vi "Two Agilent N6700 Series Configure Voltage.vi"() -> ()   [LabVIEW 2021]
doc: "Configures the power supply's output range on a channel, configures the DC voltage level, channel appears at the output connector and takes a measurement on the output signal and returns the measured value."
uses:
  <instrlib>/Agilent N6700 Series/Agilent N6700 Series.lvlib
panel:
  in  "Vin SMU":refnum<visa-resource-name>
  in  "Vin SMUChannel":string="1"
  in  "Vin Voltage Range":dbl=10.0 format="%^.3e"
  in  "Vin Voltage Level":dbl=5.0 format="%^.3e"
  out "Vin Voltage Measurement":dbl format="%^.3e"
  in  "Vin Behavior":i32(ring) items=["Regulatory Limit", "Trip Limit"]
  in  "Vin Current Limit":dbl=1.0 format="%^.3e"
  in  "error in":errorcluster {"code" format="%.0x"}
  out "error out":errorcluster {"code" format="%.0x"}
  in  "Load Current Limit":dbl=1.0 format="%^.3e"
  in  "Behavior":i32(ring) items=["Regulatory Limit", "Trip Limit"]
  out "Load Voltage Measurement":dbl format="%^.3e"
  in  "Load Voltage Level":dbl=5.0 format="%^.3e"
  in  "Load Voltage Range":dbl=10.0 format="%^.3e"
  in  "Load SMUChannel":string="1"
  in  "Load SMU":refnum<visa-resource-name>
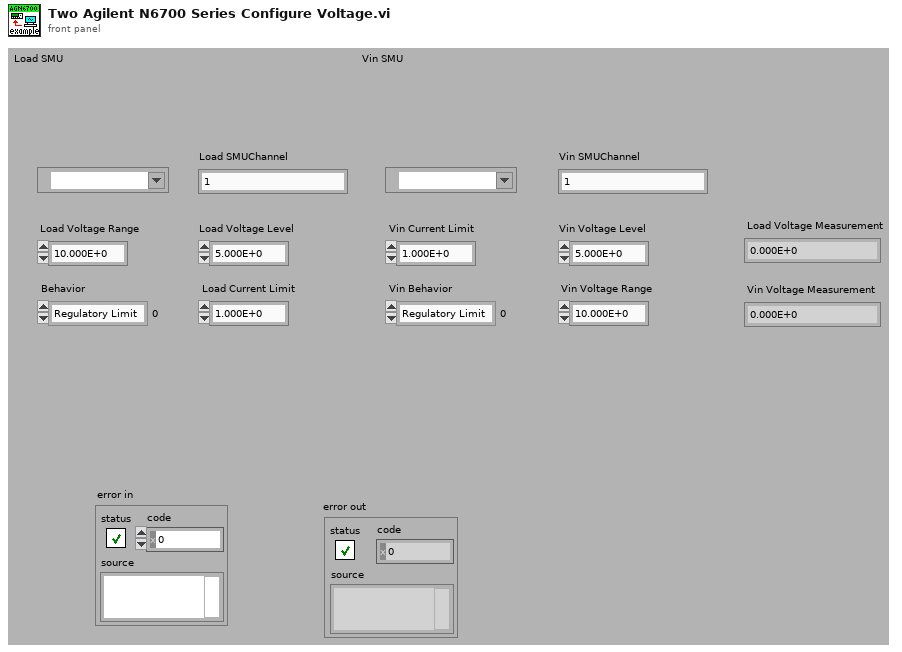
[diagram p1: front panel]
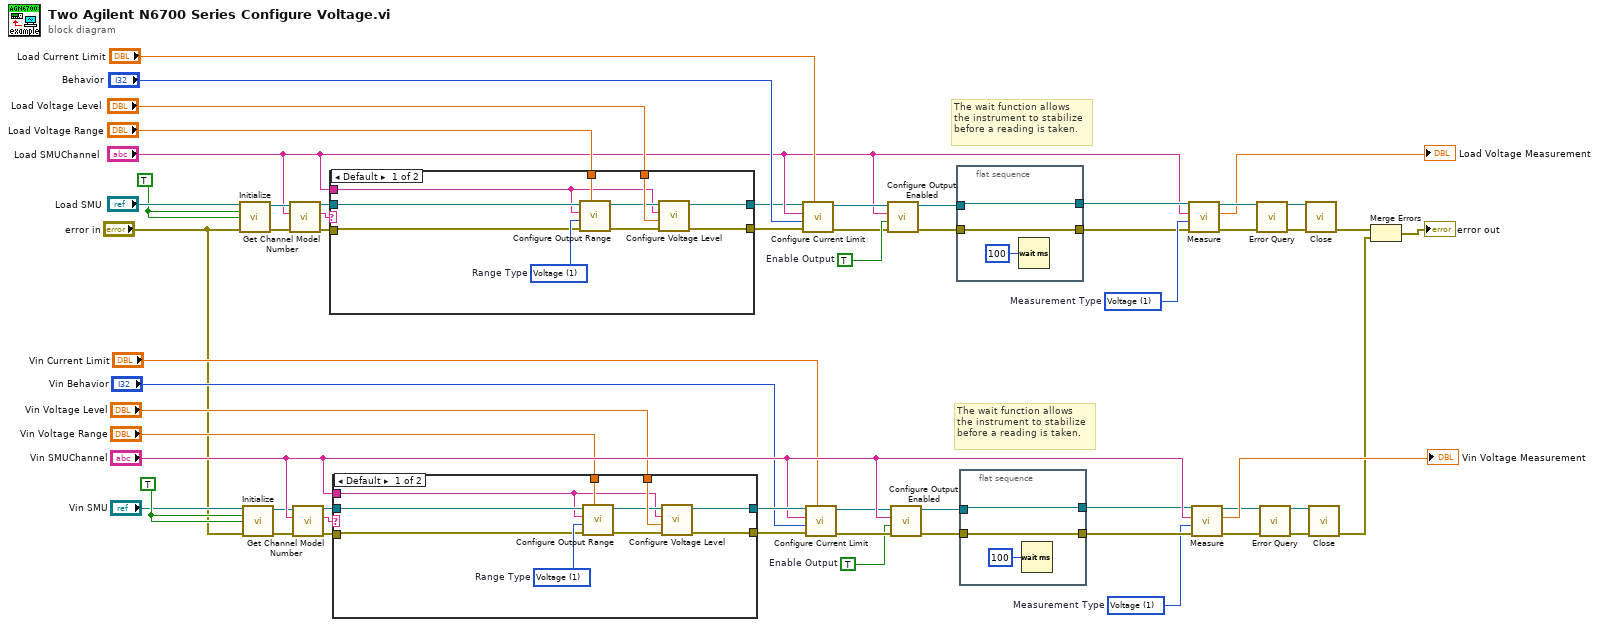
[diagram p0: block diagram]
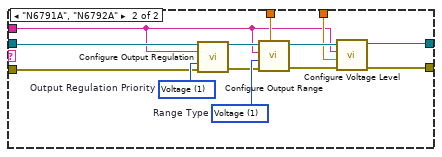
[diagram p2: hidden frame]
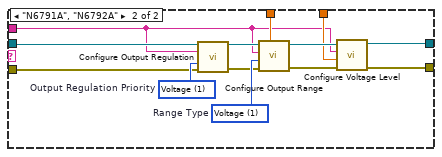
[diagram p3: hidden frame]
diagram:
  w13 = TRUE ("Reset? (T: Yes)")
  w12 = 1 items=["Voltage"=1, "Current"=0]  # Measurement Type
  w11 = TRUE  # Enable Output
  w49 = TRUE ("Reset? (T: Yes)")
  w50 = 1 items=["Voltage"=1, "Current"=0]  # Measurement Type
  w51 = TRUE  # Enable Output
  # "The wait function allows \nthe instrument to stabilize\nbefore a reading is taken."
  # "The wait function allows \nthe instrument to stabilize\nbefore a reading is taken."
  n1 = call <instrlib>:"Initialize.vi"("VISA resource name"="Load SMU", "ID Query? (T: Yes)"=w49, "Reset? (T: Yes)"=w49, "error in (no error)"="error in") -> ("VISA resource name out"=w40:refnum<visa-resource-name>, "error out"=w39:errorcluster)  [unwired: 10 in]
  n2 = call <instrlib>:"Initialize.vi"("VISA resource name"="Vin SMU", "ID Query? (T: Yes)"=w13, "Reset? (T: Yes)"=w13, "error in (no error)"="error in") -> ("VISA resource name out"=w22:refnum<visa-resource-name>, "error out"=w23:errorcluster)  [unwired: 10 in]
  n3 = call <instrlib>:"Get Channel Model Number.vi"("error in (no error)"=w39, "Channel Name (1)"="Load SMUChannel", "VISA resource name"=w40) -> ("error out"=w37:errorcluster, "Model Number"=w36:string, "VISA resource name out"=w38:refnum<visa-resource-name>)  [unwired: 6 in]
  n4 = call <instrlib>:"Get Channel Model Number.vi"("error in (no error)"=w23, "Channel Name (1)"="Vin SMUChannel", "VISA resource name"=w22) -> ("error out"=w25:errorcluster, "Model Number"=w26:string, "VISA resource name out"=w24:refnum<visa-resource-name>)  [unwired: 6 in]
  n5 = case shown="Default" w36 {
    tunnel: "Load Voltage Range" -> [w65 w81]
    tunnel: "Load SMUChannel" -> [w59 w71]
    tunnel: w38 -> [w67 w76]
    tunnel: w37 -> [w66 w75]
    tunnel: "Load Voltage Level" -> [w63 w72]
    tunnel: [w61 w69] -> w33
    tunnel: [w60 w70] -> w32
    frame Default {
      w68 = 1 items=["Voltage"=1, "Current"=0]  # Range Type
      n6 = call <instrlib>:"Configure Output Range.vi"("Range (0.0)"=w65, "error in (no error)"=w66, "Range Type (1: Voltage)"=w68, "Channel Name (1)"=w59, "VISA resource name"=w67) -> ("error out"=w64:errorcluster, "VISA resource name out"=w62:refnum<visa-resource-name>)  [unwired: 5 in]
      n7 = call <instrlib>:"Configure Voltage Level.vi"("error in (no error)"=w64, "Level  (0.0 volts)"=w63, "Channel Name (1)"=w59, "VISA resource name"=w62) -> ("error out"=w61:errorcluster, "VISA resource name out"=w60:refnum<visa-resource-name>)  [unwired: 6 in]
    }
    frame "N6791A", "N6792A" {
      w77 = 1 items=["Voltage"=1, "Current"=0]  # Output Regulation Priority
      w80 = 1 items=["Voltage"=1, "Current"=0]  # Range Type
      n8 = call <instrlib>:"Configure Output Regulation.vi"("VISA resource name"=w76, "Channel Name (1)"=w71, "Output Regulation Priority (1: Voltage)"=w77, "error in (no error)"=w75) -> ("VISA resource name out"=w79:refnum<visa-resource-name>, "error out"=w78:errorcluster)  [unwired: 10 in]
      n9 = call <instrlib>:"Configure Output Range.vi"("Range (0.0)"=w81, "error in (no error)"=w78, "Range Type (1: Voltage)"=w80, "Channel Name (1)"=w71, "VISA resource name"=w79) -> ("error out"=w73:errorcluster, "VISA resource name out"=w74:refnum<visa-resource-name>)  [unwired: 5 in]
      n10 = call <instrlib>:"Configure Voltage Level.vi"("error in (no error)"=w73, "Level  (0.0 volts)"=w72, "Channel Name (1)"=w71, "VISA resource name"=w74) -> ("error out"=w69:errorcluster, "VISA resource name out"=w70:refnum<visa-resource-name>)  [unwired: 6 in]
    }
  }
  n11 = case shown="Default" w26 {
    tunnel: "Vin Voltage Range" -> [w88 w104]
    tunnel: "Vin SMUChannel" -> [w82 w94]
    tunnel: w24 -> [w90 w99]
    tunnel: w25 -> [w89 w98]
    tunnel: "Vin Voltage Level" -> [w86 w95]
    tunnel: [w84 w92] -> w29
    tunnel: [w83 w93] -> w30
    frame Default {
      w91 = 1 items=["Voltage"=1, "Current"=0]  # Range Type
      n12 = call <instrlib>:"Configure Output Range.vi"("Range (0.0)"=w88, "error in (no error)"=w89, "Range Type (1: Voltage)"=w91, "Channel Name (1)"=w82, "VISA resource name"=w90) -> ("error out"=w87:errorcluster, "VISA resource name out"=w85:refnum<visa-resource-name>)  [unwired: 5 in]
      n13 = call <instrlib>:"Configure Voltage Level.vi"("error in (no error)"=w87, "Level  (0.0 volts)"=w86, "Channel Name (1)"=w82, "VISA resource name"=w85) -> ("error out"=w84:errorcluster, "VISA resource name out"=w83:refnum<visa-resource-name>)  [unwired: 6 in]
    }
    frame "N6791A", "N6792A" {
      w100 = 1 items=["Voltage"=1, "Current"=0]  # Output Regulation Priority
      w103 = 1 items=["Voltage"=1, "Current"=0]  # Range Type
      n14 = call <instrlib>:"Configure Output Regulation.vi"("VISA resource name"=w99, "Channel Name (1)"=w94, "Output Regulation Priority (1: Voltage)"=w100, "error in (no error)"=w98) -> ("VISA resource name out"=w102:refnum<visa-resource-name>, "error out"=w101:errorcluster)  [unwired: 10 in]
      n15 = call <instrlib>:"Configure Output Range.vi"("Range (0.0)"=w104, "error in (no error)"=w101, "Range Type (1: Voltage)"=w103, "Channel Name (1)"=w94, "VISA resource name"=w102) -> ("error out"=w96:errorcluster, "VISA resource name out"=w97:refnum<visa-resource-name>)  [unwired: 5 in]
      n16 = call <instrlib>:"Configure Voltage Level.vi"("error in (no error)"=w96, "Level  (0.0 volts)"=w95, "Channel Name (1)"=w94, "VISA resource name"=w97) -> ("error out"=w92:errorcluster, "VISA resource name out"=w93:refnum<visa-resource-name>)  [unwired: 6 in]
    }
  }
  n17 = call <instrlib>:"Configure Current Limit.vi"("Limit (0.0 amps)"="Load Current Limit", "error in (no error)"=w33, "Behavior (0: Regulatory Limit)"="Behavior", "Channel Name (1)"="Load SMUChannel", "VISA resource name"=w32) -> ("error out"=w48:errorcluster, "VISA resource name out"=w47:refnum<visa-resource-name>)  [unwired: 5 in]
  n18 = call <instrlib>:"Configure Current Limit.vi"("Limit (0.0 amps)"="Vin Current Limit", "error in (no error)"=w29, "Behavior (0: Regulatory Limit)"="Vin Behavior", "Channel Name (1)"="Vin SMUChannel", "VISA resource name"=w30) -> ("error out"=w14:errorcluster, "VISA resource name out"=w15:refnum<visa-resource-name>)  [unwired: 5 in]
  n19 = call <instrlib>:"Configure Output Enabled.vi"("error in (no error)"=w48, "Enable Output (False)"=w51, "Channel Name (1)"="Load SMUChannel", "VISA resource name"=w47) -> ("error out"=w41:errorcluster, "VISA resource name out"=w44:refnum<visa-resource-name>)  [unwired: 6 in]
  n20 = call <instrlib>:"Configure Output Enabled.vi"("error in (no error)"=w14, "Enable Output (False)"=w11, "Channel Name (1)"="Vin SMUChannel", "VISA resource name"=w15) -> ("error out"=w21:errorcluster, "VISA resource name out"=w18:refnum<visa-resource-name>)  [unwired: 6 in]
  n21 = flat-sequence {
    tunnel: w44 -> [w107]
    tunnel: [w107] -> w43
    tunnel: [w105] -> w42
    tunnel: w41 -> [w105]
    frame #0 {
      n22 = Wait (ms)(milliseconds to wait=u32 100) -> ()  [unwired: 1 out]
    }
  }
  n23 = flat-sequence {
    tunnel: w18 -> [w110]
    tunnel: [w110] -> w19
    tunnel: [w108] -> w20
    tunnel: w21 -> [w108]
    frame #0 {
      n24 = Wait (ms)(milliseconds to wait=u32 100) -> ()  [unwired: 1 out]
    }
  }
  n25 = call <instrlib>:"Measure.vi"("error in (no error)"=w42, "Measurement Type (1: Voltage)"=w50, "Channel Name (1)"="Load SMUChannel", "VISA resource name"=w43) -> ("error out"=w58:errorcluster, "Measurement"=→"Load Voltage Measurement":dbl, "VISA resource name out"=w55:refnum<visa-resource-name>)  [unwired: 5 in]
  n26 = call <instrlib>:"Measure.vi"("error in (no error)"=w20, "Measurement Type (1: Voltage)"=w12, "Channel Name (1)"="Vin SMUChannel", "VISA resource name"=w19) -> ("error out"=w4:errorcluster, "Measurement"=→"Vin Voltage Measurement":dbl, "VISA resource name out"=w7:refnum<visa-resource-name>)  [unwired: 5 in]
  n27 = call <instrlib>:"Error Query.vi"("VISA resource name"=w55, "error in (no error)"=w58) -> ("VISA resource name out"=w56:refnum<visa-resource-name>, "error out"=w57:errorcluster)  [unwired: 10 in, 2 out]
  n28 = call <instrlib>:"Error Query.vi"("VISA resource name"=w7, "error in (no error)"=w4) -> ("VISA resource name out"=w6:refnum<visa-resource-name>, "error out"=w5:errorcluster)  [unwired: 10 in, 2 out]
  n29 = call <instrlib>:"Close.vi"("VISA resource name"=w56, "error in (no error)"=w57) -> ("error out"=w31:errorcluster)  [unwired: 13 in]
  n30 = call <instrlib>:"Close.vi"("VISA resource name"=w6, "error in (no error)"=w5) -> ("error out"=w1:errorcluster)  [unwired: 13 in]
  n31 = Merge Errors(w31, w1) -> (→"error out":errorcluster)
